vi "DM GV.vi"() -> ()   [LabVIEW 2019, in "DataManagment.lvlib"]
uses:
  DataManagment.lvlib
  Intertarget communication/Command + data + response cluster.ctl
  Intertarget communication/Status + response + data cluster.ctl
  Intertarget communication/CommandResponse communication.lvlib
panel:
  in  "DM event":refnum<user-event>
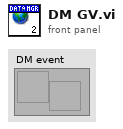
[diagram p1: front panel]
diagram:
